vi "Quick Usb Is Fpga Configured.vi"(8 "error in (no error)":errorcluster, 10 "isConfigured":u16, 11 "hDevice":u32) -> (0 "error out":errorcluster, 1 "function return":i32, 2 "isConfigured out":u16, 3 "hDevice out":u32)   [LabVIEW 2011, in "QuickUSB.lvlib"]
doc: "QUSBLIB QRETURN QuickUsbIsFpgaConfigured(\n QHANDLE hDevice, \n PQWORD isConfigured\n);"
uses:
  QuickUSB.lvlib
  QuickUSB.dll
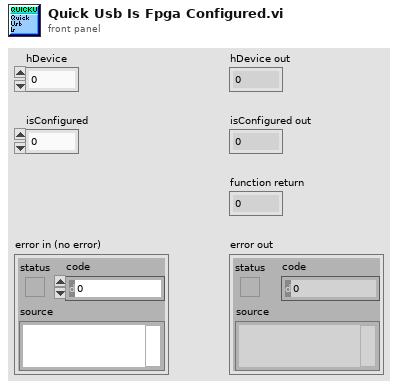
[diagram p1: front panel]
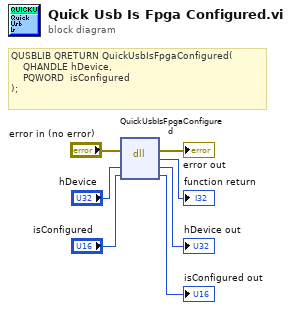
[diagram p0: block diagram]
diagram:
  # "QUSBLIB QRETURN QuickUsbIsFpgaConfigured(\n    QHANDLE hDevice, \n    PQWORD  isConfigured\n);"
  n1 = dll-call lib="C:/QuickUSB/QuickUSB.*" fn="QuickUsbIsFpgaConfigured"(error in="error in (no error)", "hDevice"="hDevice", "isConfigured"="isConfigured") -> (error out=→"error out":errorcluster, →"function return":i32, "hDevice"=→"hDevice out":u32, "isConfigured"=→"isConfigured out":u16)  [unwired: 2 in, 1 out]
